vi "SetAbortVI_popup.vi"(2 "Input Line Command":string, 3 "error in (no error)":errorcluster) -> (8 "Cancel":bool, 9 "Output Line Command":string, 10 "error out":errorcluster)   [LabVIEW 2025]
uses:
  <vilib>/Utility/error.llb/Trim Whitespace One-Sided.vi
panel:
  in  "Remote computer IP:Port":string
  in  "platform":u16(ring) items=["Mac", "PC"]
  in  "Cancel button":bool
  in  "OK Button":bool
  in  "VI name":string
  # "(empty: local host)"
  # "Case sensitive and add '.vi' at the end"
  # "For remote connection:\nGo to the VI server setting (Tools-> Options) of the server (remote) computer.\n(1) TCP/IP checked.\n(2) Verify and use the port #\n(3) Add host IP (this computer) in the Machin Access list."
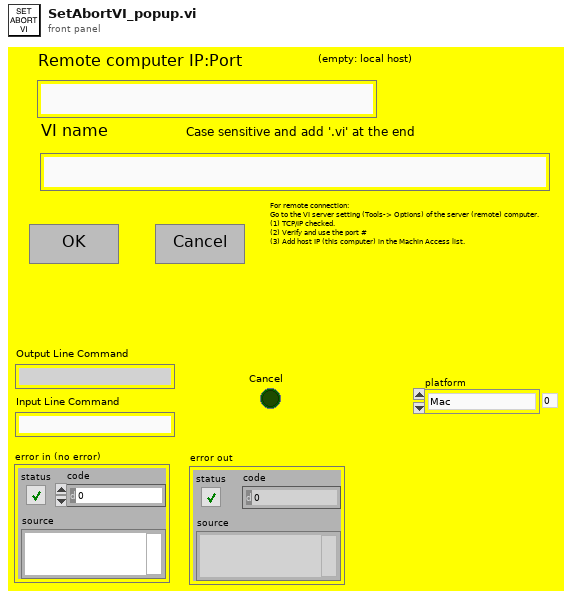
[diagram p1: front panel]
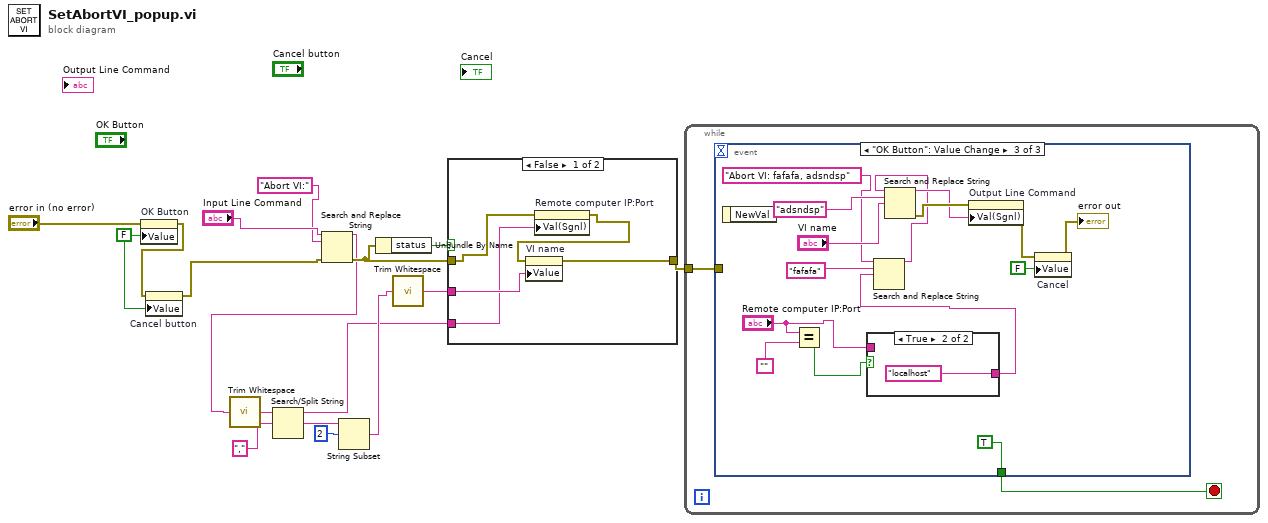
[diagram p0: block diagram]
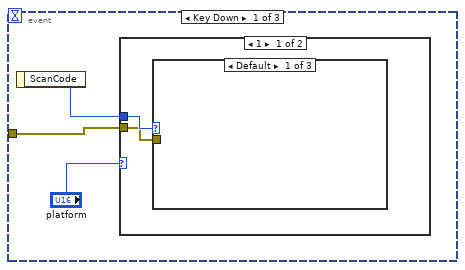
[diagram p2: hidden frame]
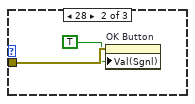
[diagram p3: hidden frame]
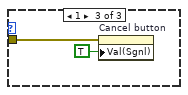
[diagram p4: hidden frame]
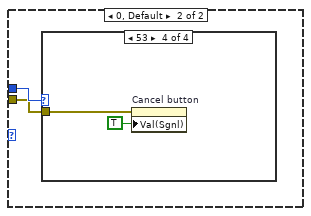
[diagram p5: hidden frame]
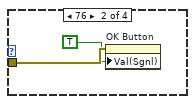
[diagram p7: hidden frame]
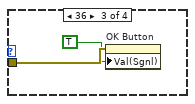
[diagram p8: hidden frame]
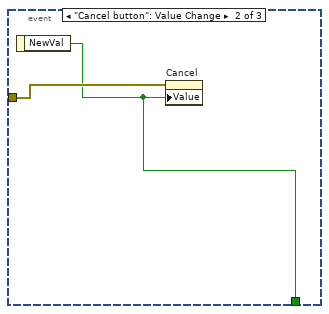
[diagram p9: hidden frame]
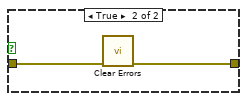
[diagram p11: hidden frame]
diagram:
  w15 = FALSE ("OK Button")
  n1 = property on="OK Button" class="Bool (strict)"(error in="error in (no error)", "Value"=w15) -> (error out=w16:errorcluster)  [unwired: 1 in, 1 out]
  n2 = property on="Cancel button" class="Bool (strict)"(error in=w16, "Value"=w15) -> (error out=w10:errorcluster)  [unwired: 1 in, 1 out]
  n3 = Search and Replace String(input string="Input Line Command", search string="Abort VI:" ("format string"), error in=w10) -> (result string=w2:string, error out=w9:errorcluster)  [unwired: 5 in, 2 out]
  n4 = call <vilib>:"Trim Whitespace.vi"("string"=w2) -> ("trimmed string"=w7:string)  [unwired: 1 in]
  n5 = Search/Split String(string=w7, search string/char (-)=",") -> (substring before match=w1:string, match + rest of string=w5:string)  [unwired: 1 in, 1 out]
  n6 = String Subset(string=w5, offset (0)=2) -> (substring=w3:string)  [unwired: 1 in]
  n7 = Unbundle By Name(w9) -> ("status"=w14:bool)
  n8 = call <vilib>:"Trim Whitespace.vi"("string"=w3) -> ("trimmed string"=w8:string)  [unwired: 1 in]
  n9 = case shown="False" w14 {
    tunnel: w9 -> [w20 w24]
    tunnel: [w22 w23] -> w13
    tunnel: w8 -> [w21 _]
    tunnel: w1 -> [w18 _]
    frame False {
      n10 = property on="Remote computer IP:Port" class="Str"(error in=w20, "Val(Sgnl)"=w18) -> (error out=w19:errorcluster)  [unwired: 1 in, 1 out]
      n11 = property on="VI name" class="Str"(error in=w19, "Value"=w21) -> (error out=w22:errorcluster)  [unwired: 1 in, 1 out]
    }
    frame True {
      n12 = call <vilib>:"Clear Errors.vi"("error in (no error)"=w24) -> ("error out"=w23:errorcluster)  [unwired: 5 in, 1 out]
    }
  }
  n13 = while {
    tunnel: w13 -> [w26]
    stop <- w25 stop-if-true
    n14 = event shown="[2] \"OK Button\": Value Change" {
      selector: _ -> [_ _ _]
      dyn-events: _ -> [_ _ _]
      timeout: _ -> [_ _ _]
      tunnel: w26 -> [w28 w45 _]
      tunnel: [_ w44 TRUE] -> w25
      event Key Down {
        n15 = event-data() -> ("ScanCode"=w29:i16)  [unwired: 1 in]
        n16 = case shown="1" "platform" {
          tunnel: w29 -> [w31 w37]
          tunnel: w28 -> [w30 w36]
          frame 1 {
            n17 = case shown="Default" w31 {
              tunnel: w30 -> [_ w33 w35]
              frame Default {
              }
              frame 28 {
                n18 = property on="OK Button" class="Bool (strict)"(error in=w33, "Val(Sgnl)"=TRUE ("Value (Signaling)")) -> ()  [unwired: 1 in, 2 out]
              }
              frame 1 {
                n19 = property on="Cancel button" class="Bool (strict)"(error in=w35, "Val(Sgnl)"=TRUE ("Value (Signaling)")) -> ()  [unwired: 1 in, 2 out]
              }
            }
          }
          frame 0, Default {
            n20 = case shown="53" w37 {
              tunnel: w36 -> [_ w39 w41 w43]
              frame Default {
              }
              frame 76 {
                n21 = property on="OK Button" class="Bool (strict)"(error in=w39, "Val(Sgnl)"=TRUE ("Value (Signaling)")) -> ()  [unwired: 1 in, 2 out]
              }
              frame 36 {
                n22 = property on="OK Button" class="Bool (strict)"(error in=w41, "Val(Sgnl)"=TRUE ("Value (Signaling)")) -> ()  [unwired: 1 in, 2 out]
              }
              frame 53 {
                n23 = property on="Cancel button" class="Bool (strict)"(error in=w43, "Val(Sgnl)"=TRUE ("Value (Signaling)")) -> ()  [unwired: 1 in, 2 out]
              }
            }
          }
        }
      }
      event "Cancel button": Value Change {
        n24 = event-data() -> ("NewVal"=w44:bool)  [unwired: 1 in]
        n25 = property on="Cancel" class="Bool (strict)"(error in=w45, "Value"=w44) -> ()  [unwired: 1 in, 2 out]
      }
      event "OK Button": Value Change {
        n26 = event-data() -> ()  [unwired: 1 in, 1 out]
        n27 = Equal?(x="Remote computer IP:Port", y="") -> (x = y?=w51:bool)
        n28 = case shown="True" w51 {
          tunnel: [w61 "localhost" ("search string")] -> w48
          tunnel: "Remote computer IP:Port" -> [w61 _]
          frame False {
          }
          frame True {
          }
        }
        n29 = Search and Replace String(input string="Abort VI: fafafa, adsndsp", search string="fafafa", replace string=w48) -> (result string=w47:string)  [unwired: 5 in, 3 out]
        n30 = Search and Replace String(input string=w47, search string="adsndsp", replace string="VI name") -> (result string=w58:string, error out=w59:errorcluster)  [unwired: 5 in, 2 out]
        n31 = property on="Output Line Command" class="Str"(error in=w59, "Val(Sgnl)"=w58) -> (error out=w56:errorcluster)  [unwired: 1 in, 1 out]
        n32 = property on="Cancel" class="Bool (strict)"(error in=w56, "Value"=FALSE ("Cancel")) -> (error out=→"error out":errorcluster)  [unwired: 1 in, 1 out]
      }
    }
  }
